vi "Find center of bounding rectangle.vi"(4 "Bounding Rect":T1={"Left"=95.0, "Top"=190.0, "Right"=105.0, "Bottom"=211.0}) -> (1 "Center (pix)":cluster{"X":i32, "Y":i32}={"X"=100, "Y"=200})   [LabVIEW 2013]
uses:
  Project Vis/Image Analysis/Analysis type defs/Bounding rectangle cluster.ctl
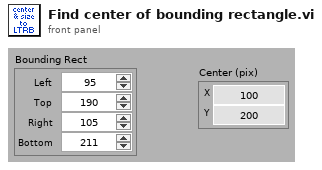
[diagram p1: front panel]
types:
  T1 = typedef "Bounding rectangle cluster.ctl" = cluster{"Left":dbl, "Top":dbl, "Right":dbl, "Bottom":dbl}
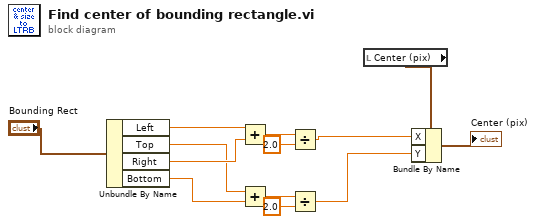
[diagram p0: block diagram]
diagram:
  n1 = Unbundle By Name("Bounding Rect") -> ("Left"=w12:dbl, "Top"=w4:dbl, "Right"=w11:dbl, "Bottom"=w3:dbl)
  n2 = Add(x=w12, y=w11) -> (x+y=w10:dbl)
  n3 = Add(x=w4, y=w3) -> (x+y=w5:dbl)
  n4 = Divide(x=w10, y=2.0) -> (x/y=w2:dbl)
  n5 = Divide(x=w5, y=2.0) -> (x/y=w1:dbl)
  n6 = local read "Center (pix)"() -> (w8:cluster{"X":i32, "Y":i32})
  n7 = Bundle By Name(cluster=w8, "X"=w2, "Y"=w1) -> (→"Center (pix)":cluster{"X":i32, "Y":i32})
